vi "my_uart.vi"() -> ()   [LabVIEW 2014]
uses:
  Program Files (x86)/National Instruments/LabVIEW 2014/examples/Instrument IO/Serial/support/Serial - Settings.ctl
  <vilib>/Instr/_visa.llb/VISA Configure Serial Port (Instr).vi
panel:
  out "字节长度":u32
  out "布尔":bool
  in  "终止符":u8=10 format="%.0x"
  in  "VISA资源名称":refnum<visa-resource-name>="COM1"
  in  "串口设置":T1={"波特率"=38400, "数据比特"=8, "奇偶"=enum."None", "停止位"=10, "流控制"=0} {"流控制" items=["无"=0, "XON/XOFF"=1, "RTS/CTS"=2, "DTR/DSR"=4]; "停止位" items=["1.0"=10, "1.5"=15, "2.0"=20]; "数据比特" min=5 max=8 step=1; "波特率" items=["75"=75, "110"=110, "134"=134, "150"=150, "300"=300, "600"=600, "1200"=1200, "1800"=1800, "2400"=2400, "4800"=4800, "7200"=7200, "9600"=9600, "14400"=14400, "19200"=19200, "28800"=28800, "38400"=38400, "56000"=56000, "57600"=57600, "115200"=115200, "128000"=128000, "230400"=230400]}
  in  "终止符时结束读取？":bool=TRUE
  in  "读数":u32=1000
  in  "停止":bool
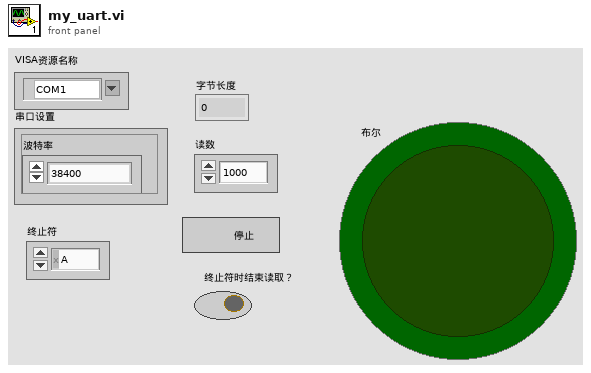
[diagram p1: front panel]
types:
  T1 = typedef "Serial - Settings.ctl" = cluster{"波特率":u32, "数据比特":u16, "奇偶":enum16{"None", "Odd", "Even", "Mark", "Space"}, "停止位":u16, "流控制":u16}
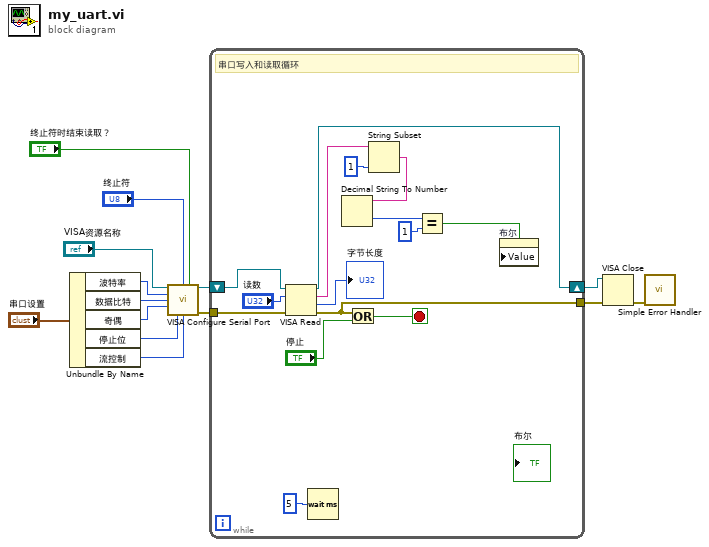
[diagram p0: block diagram]
diagram:
  n1 = Unbundle By Name("串口设置") -> ("波特率"=w10:u32, "数据比特"=w11:u16, "奇偶"=w12:enum16{"None", "Odd", "Even", "Mark", "Space"}, "停止位"=w13:u16, "流控制"=w4:u16)
  n2 = call-poly "VISA Configure Serial Port"("VISA resource name"="VISA资源名称", "termination char\n(0xA = '\\n' = LF)"="终止符", "Enable Termination\nChar (T)"="终止符时结束读取？", "baud rate (9600)"=w10, "data bits (8)"=w11, "parity (0:none)"=w12, "stop bits (10: 1 bit)"=w13, "flow control (0:none)"=w4) -> ("VISA resource name out"=w2:refnum<visa-resource-name>, "error out"=w1:errorcluster)  [unwired: 2 in, 4 out]
  n3 = while {
    shift-right: [w29] -> w5
    shift-left: w2 -> [w24]
    tunnel: w1 -> [w23]
    tunnel: [w26] -> w6
    stop <- w27 stop-if-true
    # "串口写入和读取循环"
    n4 = VISA Read(VISA resource name=w24, byte count="读数", error in (no error)=w23) -> (VISA resource name out=w29:refnum<visa-resource-name>, read buffer=w20:string, return count=→"字节长度":u32, error out=w26:errorcluster)
    n5 = Wait (ms)(milliseconds to wait=u32 5) -> ()  [unwired: 1 out]
    n6 = Or(x=w26, y="停止") -> (x .or. y?=w27:bool)
    n7 = String Subset(string=w20, length (rest)=1 ("长度（剩余）")) -> (substring=w18:string)  [unwired: 1 in]
    n8 = Decimal String To Number(string=w18) -> (number=w17:i32)  [unwired: 2 in, 1 out]
    n9 = Equal?(x=w17, y=1) -> (x = y?=w15:bool)
    n10 = property on="布尔" class="Bool (严格)"("Value"=w15) -> ()  [unwired: 2 in, 2 out]
  }
  n11 = VISA Close(VISA resource name=w5, error in (no error)=w6) -> (error out=w7:errorcluster)
  n12 = call <vilib>:"Simple Error Handler.vi"("error in (no error)"=w7) -> ()  [unwired: 1 in, 8 out]
